vi "z[Lambda_tau,T,W,t_0]_Analytical.vi"(6 "t0":ext, 7 "Harmonic f":ext, 9 "W":ext, 10 "T":ext, 11 "tau":ext) -> (3 "z":cxt)   [LabVIEW 2021, in "Phasor.lvlib"]
uses:
  Phasor.lvlib
  Math/ix/ix (EXT).vi
  Math/Math.lvlib
  7f9257a1-fee9-4441-afd6-b067f301fbb6.vi
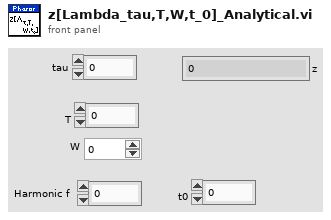
[diagram p1: front panel]
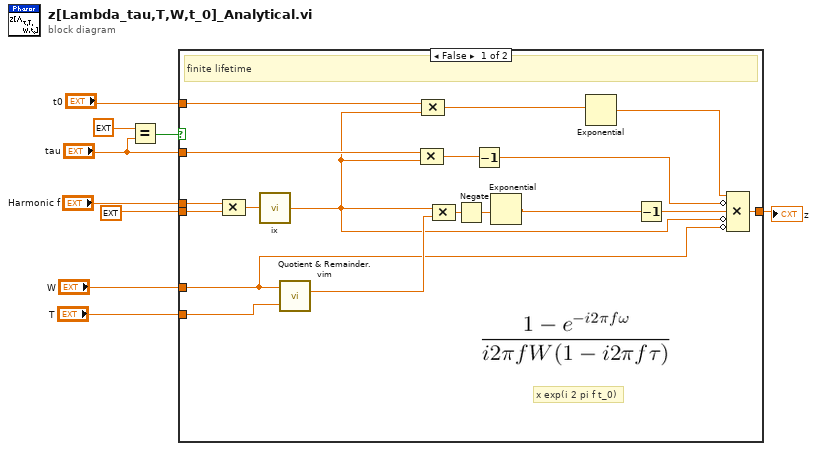
[diagram p0: block diagram]
diagram:
  n1 = Equal?(x=ext inf ("y"), y="tau") -> (x = y?=w2:bool)
  n2 = case shown="False" w2 {
    tunnel: "Harmonic f" -> [w27 _]
    tunnel: "T" -> [w10 _]
    tunnel: ext 6.283185307179586477 -> [w26 _]
    tunnel: "W" -> [w21 _]
    tunnel: [w17 _] -> w6
    tunnel: "t0" -> [w16 _]
    tunnel: "tau" -> [w13 _]
    frame False {
      # "x exp(i 2 pi f t_0)"
      # "finite lifetime"
      n3 = Compound Arithmetic op=MULTIPLY(w27, w26) -> (w12:ext)
      n4 = call-poly "ix.vi"("x (1)"=w12) -> ("i.(x)"=w11:cxt)
      n5 = call "Quotient & Remainder.vim"("y"=w10, "x"=w21) -> ("x - E(x/y)y"=w24:ext)  [unwired: 1 out]
      n6 = Compound Arithmetic op=MULTIPLY(w13, w11) -> (w19:cxt)
      n7 = Compound Arithmetic op=MULTIPLY(w16, w11) -> (w15:cxt)
      n8 = Compound Arithmetic op=MULTIPLY(w11, w24) -> (w25:cxt)
      n9 = Negate(x=w25) -> (-x=w23:cxt)
      n10 = Decrement(x=w19) -> (x-1=w18:cxt)
      n11 = Exponential(1:w23) -> (0:w22:cxt)
      n12 = Exponential(1:w15) -> (0:w14:cxt)
      n13 = Decrement(x=w22) -> (x-1=w20:cxt)
      n14 = Compound Arithmetic op=MULTIPLY(w14, invert w18, w20, invert w11, invert w21) -> (w17:cxt)
    }
    frame True {
      # "infinite lifetime"
    }
  }
  "z" <- w6
